vi "UnicNameFinder.vi"(1 "Array":T1[](array[typedef])) -> (0 "String":string)   [LabVIEW 2014]
uses:
  TempConfig.ctl
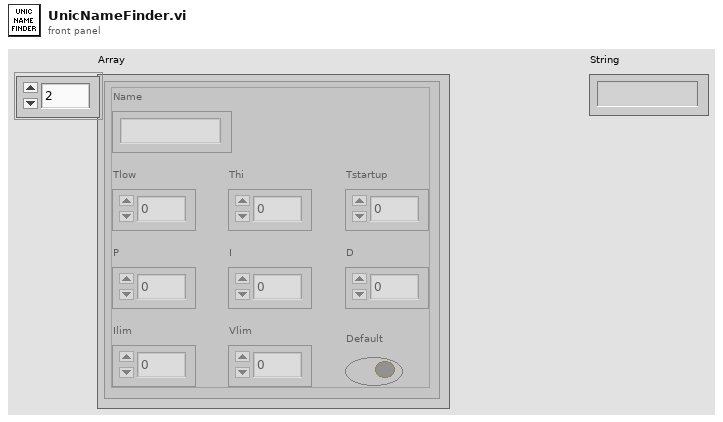
[diagram p1: front panel]
types:
  T1 = typedef "TempConfig.ctl" = cluster{"Name":string, "Thi":dbl, "Tlow":dbl, "Tstartup":dbl, "P":dbl, "I":dbl, "D":dbl, "Ilim":dbl, "Vlim":dbl, "Default":bool}
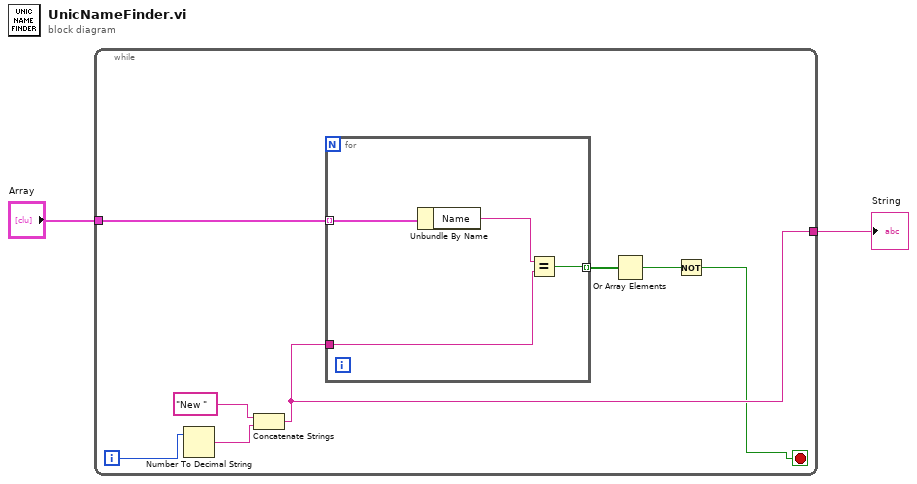
[diagram p0: block diagram]
diagram:
  n1 = while {
    tunnel: "Array" -> [w7]
    tunnel: [w6] -> w1
    i -> [w10]
    stop <- w3 stop-if-true
    n2 = Number To Decimal String(number=w10) -> (decimal integer string=w8:string)  [unwired: 1 in]
    n3 = Concatenate Strings("New ", w8) -> (w6:string)
    n4 = for {
      tunnel: w6 -> [w12]
      tunnel: w7 -> [w14] mode=indexing
      tunnel: [w11] -> w5 mode=indexing
      n5 = Unbundle By Name(w14) -> ("Name"=w13:string)
      n6 = Equal?(x=w13, y=w12) -> (x = y?=w11:bool)
    }
    n7 = Or Array Elements(Boolean array=w5) -> (logical OR=w4:bool)
    n8 = Not(x=w4) -> (.not. x?=w3:bool)
  }
  "String" <- w1
